vi "Check DB Connection.vi"(8 "Error In":errorcluster, 10 "Connection String":string) -> (0 "Error Out":errorcluster, 3 "OK":bool)   [LabVIEW 2015]
doc: "Checks for a database connection at the UDL file you specify.\n\nCopyright © 2010 Blue Ridge Test, Inc.\nwww.BlueRidgeTest.com"
panel:
  in  "ADODB._Connection":refnum<k7>
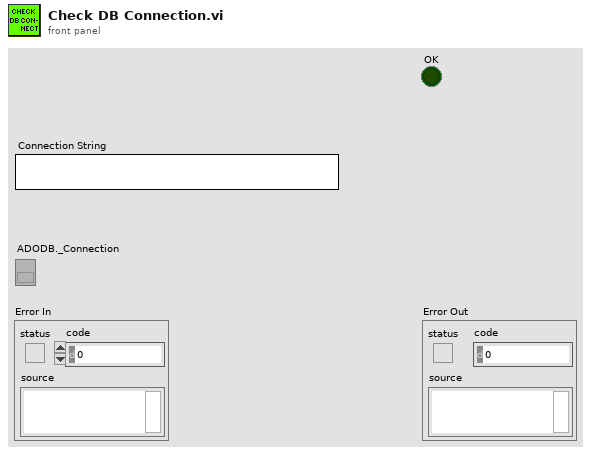
[diagram p1: front panel]
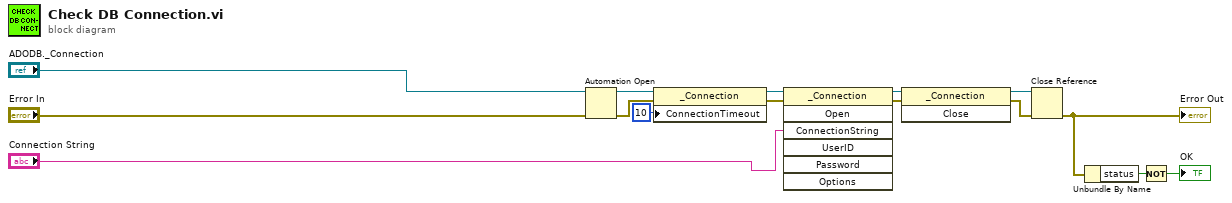
[diagram p0: block diagram]
diagram:
  n1 = Automation Open(error in (no error)="Error In", Automation Refnum="ADODB._Connection") -> (Automation Refnum=w8:refnum<k7>, error out=w7:errorcluster)  [unwired: 2 out]
  n2 = property class="_Connection"(reference=w8, error in=w7, "ConnectionTimeout"=10) -> (reference out=w10:refnum<k7>, error out=w11:errorcluster)
  n3 = invoke class="_Connection" method="Open"(reference=w10, error in=w11, "ConnectionString"="Connection String") -> (reference out=w13:refnum<k7>, error out=w12:errorcluster)  [unwired: 4 in, 5 out]
  n4 = invoke class="_Connection" method="Close"(reference=w13, error in=w12) -> (reference out=w14:refnum<k7>, error out=w15:errorcluster)  [unwired: 1 in, 1 out]
  n5 = Close Reference(reference=w14, error in (no error)=w15) -> (error out=w4:errorcluster)
  "Error Out" <- w4
  n6 = Unbundle By Name(w4) -> ("status"=w3:bool)
  n7 = Not(x=w3) -> (.not. x?=→"OK":bool)
